vi "Actor Core.vi"(8 "error in":errorcluster, 11 "Result Info in":refnum<class "Result Info.lvclass">) -> (0 "error out":errorcluster, 3 "Actor out":refnum<class "Actor.lvclass">)   [LabVIEW 2023, in "Data Analysis.lvlib" / "Result Info.lvlib" / "Result Info.lvclass"]
doc: "(<B>Filename</B>: Actor Framework.lvlib:Actor.lvclass:Actor Core.vi)\n\nReceives messages to the actor, reacts to them, and initiates any error handling that may shut the actor down.\n\nDescendant classes may override this VI to append parallel tasks for the actor to complete while it handles messages. Overrides use the Call Parent Class Method node."
uses:
  Result Info.lvclass
  C:/Program Files/National Instruments/LabVIEW 2023/vi.lib/ActorFramework/Actor/Actor.lvclass
  <vilib>/ActorFramework/Actor/Actor.lvclass
  <vilib>/ActorFramework/Actor/Actor.lvclass/Actor.ctl
  <vilib>/ActorFramework/Message Enqueuer/Message Enqueuer.lvclass/Message Enqueuer.ctl
  Subpanel-Abstract Messages/Insert SP Msg/Insert SP Msg.lvclass/Insert SP Msg.ctl
  <vilib>/ActorFramework/Message Enqueuer/Init from Existing Queue.vi
  <vilib>/ActorFramework/Message Enqueuer/Enqueue.vi
  Subpanel-Abstract Messages/Insert SP Msg/Insert SP Msg.lvclass
  C:/Program Files/National Instruments/LabVIEW 2023/vi.lib/ActorFramework/Message/Message.lvclass
  <vilib>/ActorFramework/Message Priority Queue/Priority Enqueue.vi
  <vilib>/ActorFramework/Message Enqueuer/Message Enqueuer.lvclass
  Subpanel-Abstract/Subpanel-Abstract.lvclass
  Result Info.lvclass/Result Info.ctl
panel:
  out "version":string
  in  "Boolean":bool
  out "Boolean Out":bool
  in  "Stop":bool
  # "For assistance, please contact:\n\nAbhay Kumar at abhay.kumar@vitesco.com  \nMarywin Baskaran at marywin.baskaran@vitesco.com"
  # "Designed and Developed by"
  # "LTT\nDATA ANALYSER"
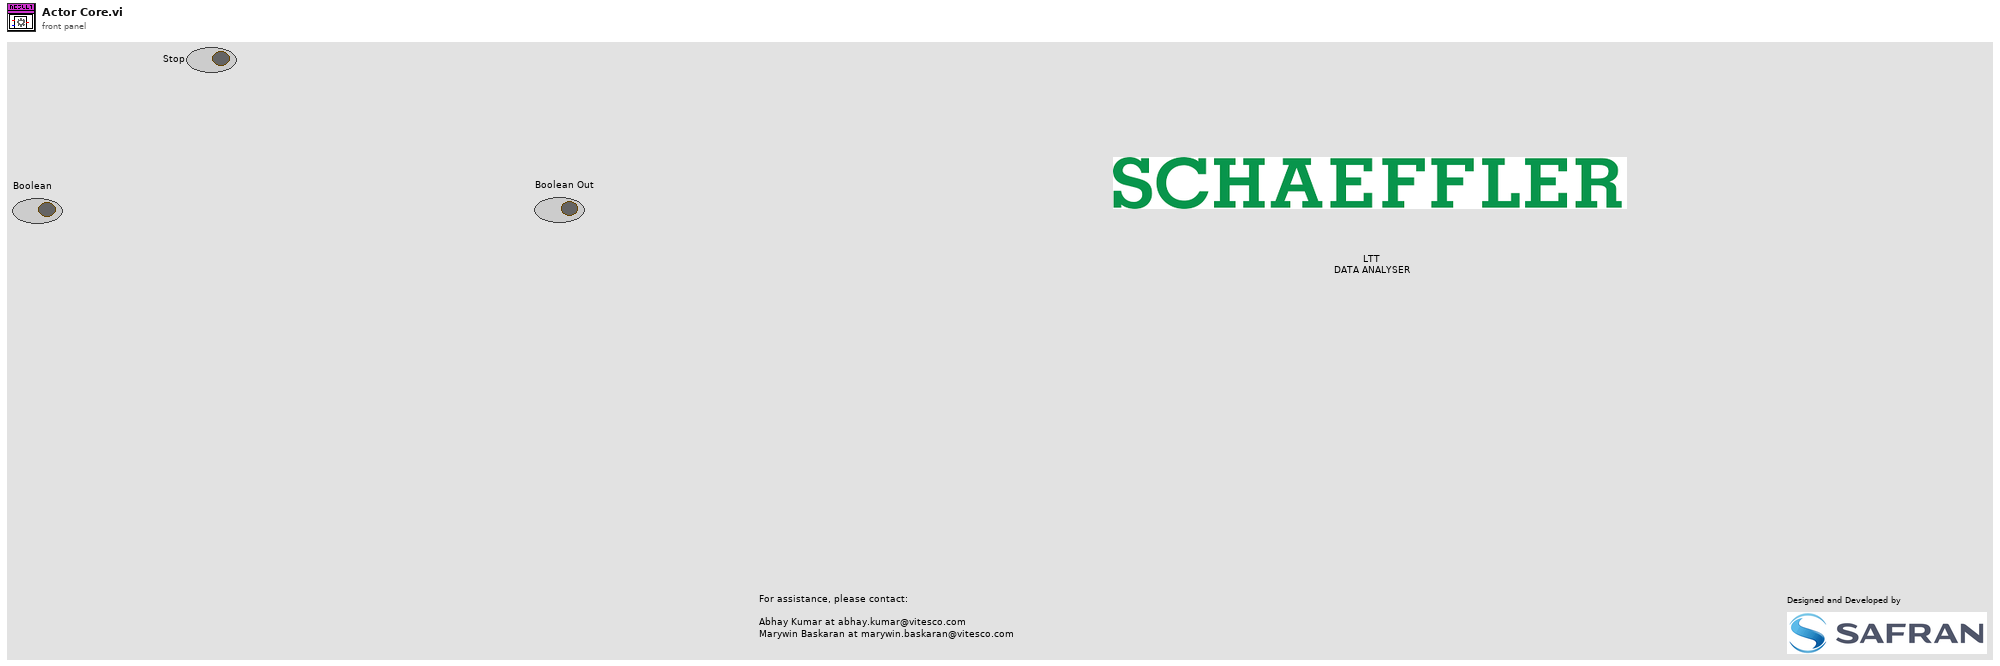
[diagram p1: front panel]
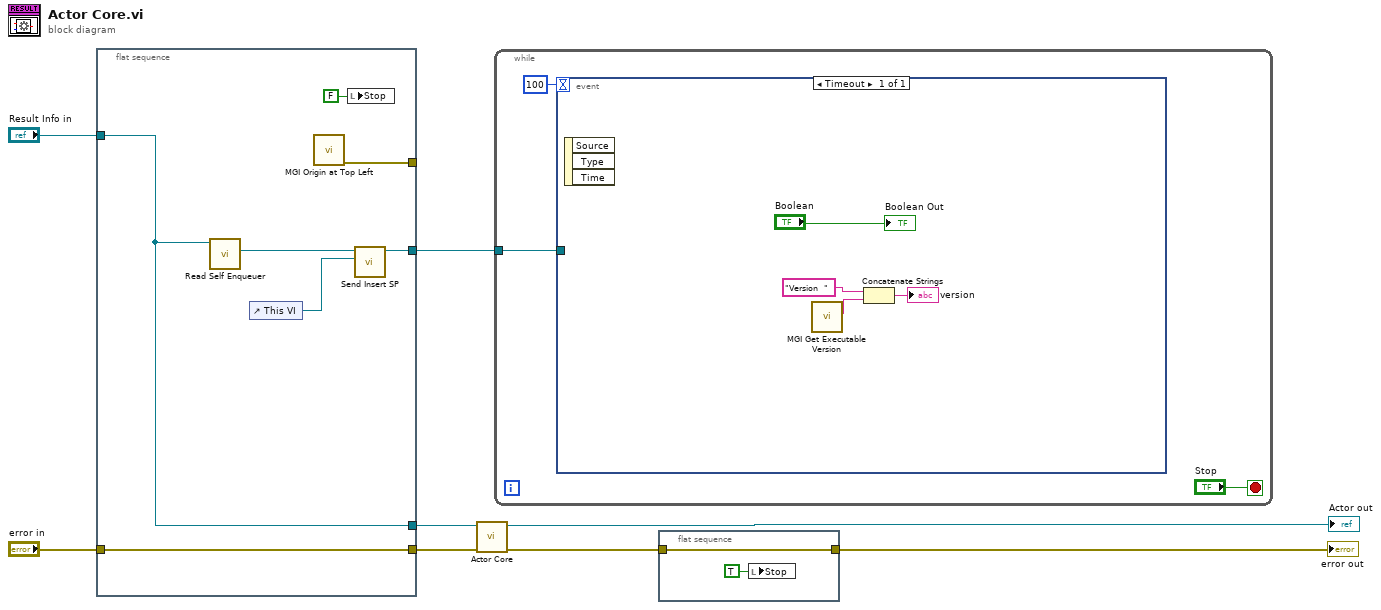
[diagram p0: block diagram]
diagram:
  n1 = flat-sequence {
    tunnel: "error in" -> [w15]
    tunnel: [w15] -> w4
    tunnel: "Result Info in" -> [w13]
    tunnel: [w13] -> w2
    tunnel: [w11] -> w1
    tunnel: [w9] -> _
    frame #0 {
      n2 = call <vilib>:"Read Self Enqueuer.vi"("Actor"=w13) -> ("Self Enqueuer"=w12:refnum<class "Message Enqueuer.lvclass">)  [unwired: 10 in]
      n3 = control-ref of="This VI"() -> (w10:refnum<vi>)
      n4 = call <userlib>:"MGI Origin at Top Left.vi"() -> ("Error Out"=w9:errorcluster)  [unwired: 9 in, 1 out]
      n5 = local write "Stop"(FALSE ("Stop")) -> ()
      n6 = call "Send Insert SP.vi"("VI Ref"=w10, "Message Enqueuer"=w12) -> ("Message Enqueuer out"=w11:refnum<class "Message Enqueuer.lvclass">)  [unwired: 8 in, 1 out]
    }
  }
  n7 = call-parent "Actor Core.vi"("error in"=w4, "Actor in"=w2) -> ("error out"=w7:errorcluster, "Actor out"=→"Actor out":refnum<class "Actor.lvclass">)  [unwired: 8 in]
  n8 = while {
    tunnel: w1 -> [w16]
    stop <- "Stop" stop-if-true
    n9 = event shown="[0] Timeout" {
      selector: _ -> [_]
      dyn-events: _ -> [_]
      timeout: 100 -> [_]
      tunnel: w16 -> [_]
      event Timeout {
        n10 = event-data() -> ()  [unwired: 1 in, 3 out]
        n11 = call <userlib>:"MGI Get Executable Version.vi"() -> ("Version"=w21:string)  [unwired: 7 in]
        n12 = Concatenate Strings("Version  " ("string"), w21) -> (→"version":string)
        "Boolean Out" <- "Boolean"
      }
    }
  }
  n13 = flat-sequence {
    tunnel: w7 -> [w24]
    tunnel: [w24] -> w6
    frame #0 {
      n14 = local write "Stop"(TRUE ("Stop")) -> ()
    }
  }
  "error out" <- w6
